vi "Play with rts cts quectel.vi"(8 "error in (no error)":errorcluster) -> (0 "error out":errorcluster, 1 "RTS control ok?":bool, 3 "PassFail":string, 4 "Comport responsive?":bool, 5 "Comport unresponsive?":bool)   [LabVIEW 2013]
uses:
  Test Globals/Global 1.vi
panel:
  out "CTS asserted? 2":bool
  out "CTS asserted?":bool
  out "VISA resource name out":refnum<visa-resource-name>
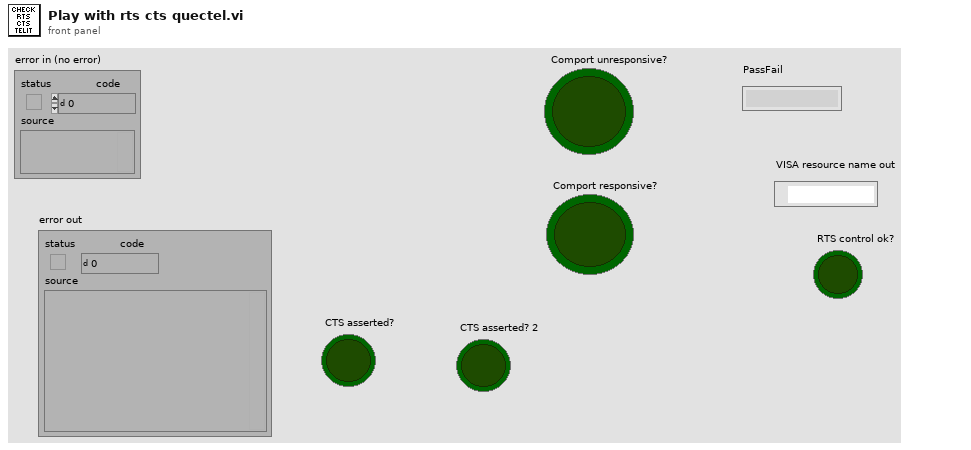
[diagram p1: front panel]
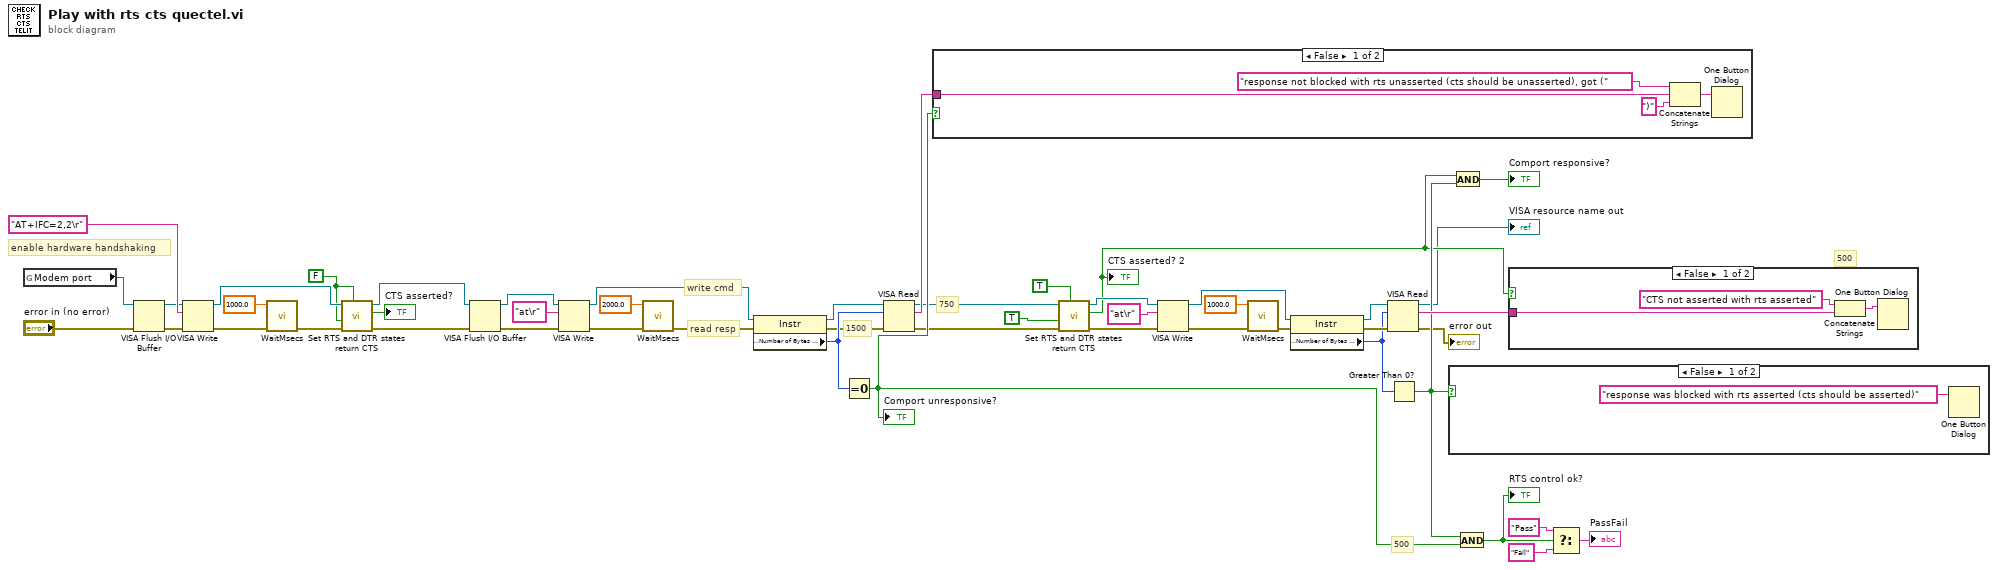
[diagram p0: block diagram]
diagram:
  w21 = FALSE ("Assert RTS?")
  # "500"
  # "500"
  # "750"
  # "1500"
  # "enable hardware handshaking"
  # "read resp"
  # "write cmd"
  n1 = global read "Global 1.vi" "Modem port"() -> (w32:refnum<visa-resource-name>)
  n2 = VISA Flush I/O Buffer(VISA resource name=w32, error in (no error)="error in (no error)") -> (VISA resource name out=w31:refnum<visa-resource-name>, error out=w30:errorcluster)  [unwired: 1 in]
  n3 = VISA Write(VISA resource name=w31, write buffer="AT+IFC=2,2\r", error in (no error)=w30) -> (VISA resource name out=w22:refnum<visa-resource-name>, error out=w9:errorcluster)  [unwired: 1 out]
  n4 = call "WaitMsecs.vi"("error in (no error)"=w9, "Wait Msecs"=1000.0) -> ("error out"=w7:errorcluster)  [unwired: 9 in]
  n5 = call "Set RTS and DTR states return CTS.vi"("Assert DTR?"=w21, "error in (no error)"=w7, "Assert RTS?"=w21, "VISA Refnum in"=w22) -> ("error out"=w3:errorcluster, "CTS asserted?"=→"CTS asserted?":bool, "Visa ref out"=w5:refnum<visa-resource-name>)  [unwired: 5 in]
  n6 = VISA Flush I/O Buffer(VISA resource name=w5, error in (no error)=w3) -> (VISA resource name out=w4:refnum<visa-resource-name>, error out=w6:errorcluster)  [unwired: 1 in]
  n7 = VISA Write(VISA resource name=w4, write buffer="at\r", error in (no error)=w6) -> (VISA resource name out=w28:refnum<visa-resource-name>, error out=w34:errorcluster)  [unwired: 1 out]
  n8 = call "WaitMsecs.vi"("error in (no error)"=w34, "Wait Msecs"=2000.0) -> ("error out"=w29:errorcluster)  [unwired: 9 in]
  n9 = property class="Instr"(reference=w28, error in=w29) -> (reference out=w37:refnum<visa-resource-name>, error out=w20:errorcluster, "Serial Settings:Number of Bytes at Serial Port"=w48:u32)
  n10 = Equal To 0?(x=w48) -> (x = 0?=w19:bool)
  "Comport unresponsive?" <- w19
  n11 = VISA Read(VISA resource name=w37, byte count=w48, error in (no error)=w20) -> (VISA resource name out=w17:refnum<visa-resource-name>, read buffer=w25:string, error out=w18:errorcluster)  [unwired: 1 out]
  n12 = case shown="False" w19 {
    tunnel: w25 -> [w52 _]
    frame False {
      n13 = Concatenate Strings("response not blocked with rts unasserted (cts should be unasserted), got (" ("message"), w52, ")" ("string")) -> (w50:string)
      n14 = One Button Dialog(message=w50) -> ()  [unwired: 1 in, 1 out]
    }
    frame True {
    }
  }
  n15 = call "Set RTS and DTR states return CTS.vi"("Assert DTR?"=TRUE, "error in (no error)"=w18, "Assert RTS?"=TRUE, "VISA Refnum in"=w17) -> ("error out"=w13:errorcluster, "CTS asserted?"=w10:bool, "Visa ref out"=w14:refnum<visa-resource-name>)  [unwired: 5 in]
  "CTS asserted? 2" <- w10
  n16 = VISA Write(VISA resource name=w14, write buffer="at\r", error in (no error)=w13) -> (VISA resource name out=w36:refnum<visa-resource-name>, error out=w11:errorcluster)  [unwired: 1 out]
  n17 = call "WaitMsecs.vi"("error in (no error)"=w11, "Wait Msecs"=1000.0) -> ("error out"=w46:errorcluster)  [unwired: 9 in]
  n18 = property class="Instr"(reference=w36, error in=w46) -> (reference out=w35:refnum<visa-resource-name>, error out=w44:errorcluster, "Serial Settings:Number of Bytes at Serial Port"=w42:u32)
  n19 = VISA Read(VISA resource name=w35, byte count=w42, error in (no error)=w44) -> (VISA resource name out=→"VISA resource name out":refnum<visa-resource-name>, read buffer=w27:string, error out=→"error out":errorcluster)  [unwired: 1 out]
  n20 = Greater Than 0?(x=w42) -> (x > 0?=w24:bool)
  n21 = case shown="False" w24 {
    frame False {
      n22 = One Button Dialog(message="response was blocked with rts asserted (cts should be asserted)") -> ()  [unwired: 1 in, 1 out]
    }
    frame True {
    }
  }
  n23 = And(x=w10, y=w24) -> (x .and. y?=→"Comport responsive?":bool)
  n24 = And(x=w24, y=w19) -> (x .and. y?=w23:bool)
  "RTS control ok?" <- w23
  n25 = case shown="False" w10 {
    tunnel: w27 -> [w56 _]
    frame False {
      n26 = Concatenate Strings("CTS not asserted with rts asserted" ("message"), w56) -> (w55:string)
      n27 = One Button Dialog(message=w55) -> ()  [unwired: 1 in, 1 out]
    }
    frame True {
    }
  }
  n28 = Select(t="Pass", s=w23, f="Fail") -> (s? t:f=→"PassFail":string)
